vi "RingNameChange.vi"(7 "PlotToDelete":i32, 8 "Enum":enum16{"Add", "Delete", "Clean"}(ring), 9 "Data aquired?":bool, 10 "name (change?)":string, 11 "PlotNumber":dbl) -> (3 "Strings&Arrays":T1(array[cluster]))   [LabVIEW 2020]
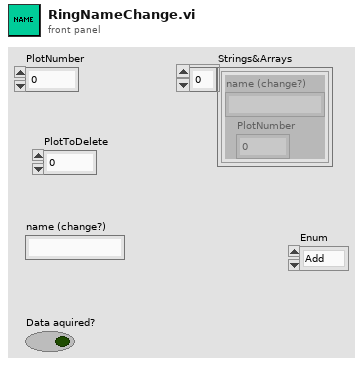
[diagram p1: front panel]
types:
  T1 = cluster{"name (change?)":string, "PlotNumber":dbl}[]
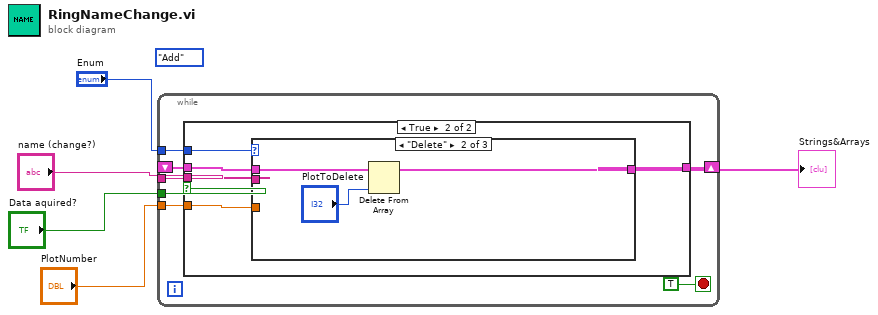
[diagram p0: block diagram]
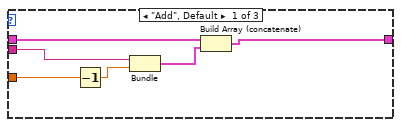
[diagram p3: hidden frame]
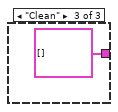
[diagram p4: hidden frame]
diagram:
  (unwired) enum16{"Add", "Delete", "Clean"}."Add"
  n1 = while {
    tunnel: "Data aquired?" -> [w12]
    shift-right: [w9] -> w2
    shift-left: _ -> [w10]
    tunnel: "name (change?)" -> [w8]
    tunnel: "PlotNumber" -> [w7]
    tunnel: "Enum" -> [w6]
    stop <- TRUE stop-if-true
    n2 = case shown="True" w12 {
      tunnel: w10 -> [w13 w18]
      tunnel: [w13 w17] -> w9
      tunnel: w8 -> [_ w16]
      tunnel: w7 -> [_ w15]
      tunnel: w6 -> [_ w14]
      frame False {
      }
      frame True {
        n3 = case shown="\"Delete\"" w14 {
          tunnel: w18 -> [w24 w27 _]
          tunnel: [w23 w25 cluster{"name (change?)":string, dbl}[] []] -> w17
          tunnel: w16 -> [w22 _ _]
          tunnel: w15 -> [w20 _ _]
          frame "Add", Default {
            n4 = Decrement(x=w20) -> (x-1=w19:dbl)
            n5 = Bundle("name (change?)"=w22, w19) -> (w21:cluster{"name (change?)":string, dbl})  [unwired: 1 in]
            n6 = Build Array (concatenate)(w24, w21) -> (w23:cluster{"name (change?)":string, dbl}[])
          }
          frame "Delete" {
            n7 = Delete From Array(array=w27, index="PlotToDelete") -> (array with subset deleted=w25:cluster{"name (change?)":string, dbl}[])  [unwired: 1 in, 1 out]
          }
          frame "Clean" {
          }
        }
      }
    }
  }
  "Strings&Arrays" <- w2
